vi "MulticolumnListbox - select all.vi"(7 "MulticolumnListbox":refnum<vi>) -> ()   [LabVIEW 2017, in "util.lvlib"]
uses:
  util.lvlib
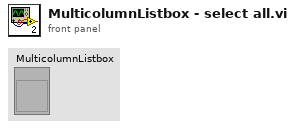
[diagram p1: front panel]
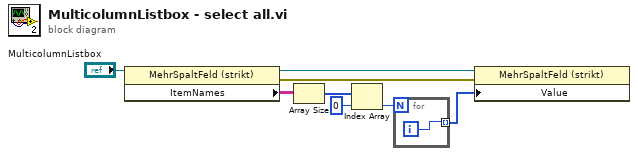
[diagram p0: block diagram]
diagram:
  n1 = property on="Eigenschaftsknoten" class="MehrSpaltFeld (strikt)"(reference="MulticolumnListbox") -> (reference out=w4:refnum<vi>, error out=w3:errorcluster, "ItemNames"=w7:string[][])  [unwired: 1 in]
  n2 = Array Size(array=w7) -> (size(s)=w6:i32[])
  n3 = Index Array(array=w6, index=0 ("Index")) -> (element=w2:i32)
  n4 = for {
    N: w2 -> [_]
    tunnel: [w9] -> w1 mode=indexing
    i -> [w9]
  }
  n5 = property on="Eigenschaftsknoten" class="MehrSpaltFeld (strikt)"(reference=w4, error in=w3, "Value"=w1) -> ()  [unwired: 2 out]
